vi "SimpleStreamingExample.vi"() -> ()   [LabVIEW 2016]
doc: "This example VI demonstrates the establishment and use of streaming peaks data from Hyperion instruments."
uses:
  h.Library/ACQ/CTL/h.ACQ.PeaksData.ctl
  h.Library/ACQ/CTL/h.ACQ.PeaksWvl.ctl
  h.Library/COMM/CTL/h.COMM.Socket Type.ctl
  h.Library.lvlib
panel:
  out "Peaks Data":T1 {"Peaks Wvls, nm"."Peak Wvls, nm" format="%#_8g"}
  out "Error":errorcluster
  in  "stop":bool
  in  "Data Rate Divider":i32=1 min=1 step=1
  in  "Address":string="10.0.0.55"
  # "Hyperion Simple Streaming Example"
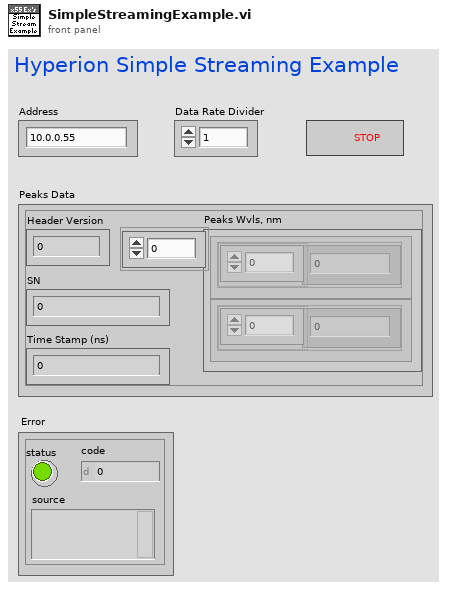
[diagram p1: front panel]
types:
  T1 = typedef "h.Library.lvlib/h.ACQ.PeaksData.ctl" = cluster{"SN":u64, "Time Stamp (ns)":u64, "Header Version":u16, "Peaks Wvls, nm":T2[]}
  T2 = typedef "h.Library.lvlib/h.ACQ.PeaksWvl.ctl" = cluster{"Peak Wvls, nm":dbl[]}
  T3 = typedef "h.Library.lvlib/h.COMM.Socket Type.ctl" = u16
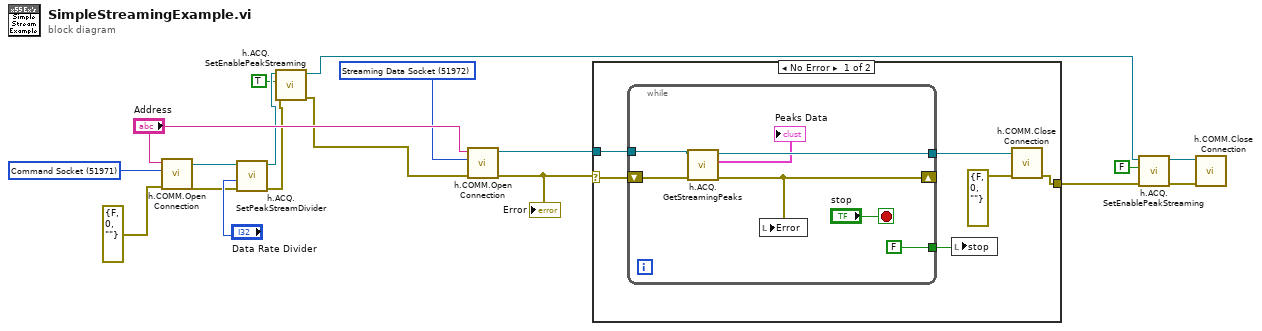
[diagram p0: block diagram]
diagram:
  w10 = T3 51972 items=["Command Socket"=51971, "Streaming Data Socket"=51972] ("Port")
  w11 = T3 51971 items=["Command Socket"=51971, "Streaming Data Socket"=51972] ("Port")
  n1 = call "h.COMM.Open Connection.vi"("error in"=errorcluster {"status"=FALSE, "code"=0, "source"=""}, "Port"=w11, "Address"="Address") -> ("error out"=w15:errorcluster, "Connection ID"=w17:refnum<k5>)  [unwired: 7 in]
  n2 = call "h.ACQ.SetPeakStreamDivider.vi"("error in"=w15, "Data Rate Divider"="Data Rate Divider", "Connection ID In"=w17) -> ("error out"=w7:errorcluster, "Connection ID Out"=w9:refnum<k5>)  [unwired: 7 in]
  n3 = call "h.ACQ.SetEnablePeakStreaming.vi"("error in"=w7, "Enable"=TRUE, "Connection ID in"=w9) -> ("error out"=w6:errorcluster, "Connection ID out"=w3:refnum<k5>)  [unwired: 7 in]
  n4 = call "h.COMM.Open Connection.vi"("error in"=w6, "Port"=w10, "Address"="Address") -> ("error out"=w13:errorcluster, "Connection ID"=w12:refnum<k5>)  [unwired: 7 in]
  "Error" <- w13
  n5 = case shown="No Error" w13 {
    selector: w13 -> [w23 _]
    tunnel: w12 -> [w20 _]
    tunnel: [w19 _] -> w4
    frame No Error {
      n6 = while {
        tunnel: [w30] -> w24
        shift-right: [w28] -> _
        shift-left: w23 -> [w29]
        tunnel: [FALSE ("stop")] -> w21
        tunnel: w20 -> [w25]
        stop <- "stop" stop-if-true
        n7 = call "h.ACQ.GetStreamingPeaks.vi"("error in"=w29, "Connection ID In"=w25) -> ("error out"=w28:errorcluster, "Peaks Data"=→"Peaks Data":T1, "Connection ID Out"=w30:refnum<k5>)  [unwired: 7 in]
        n8 = local write "Error"(w28) -> ()
      }
      n9 = local write "stop"(w21) -> ()
      n10 = call "h.COMM.Close Connection.vi"("error in"=errorcluster {"status"=FALSE, "code"=0, "source"=""}, "Connection ID"=w24) -> ("error out"=w19:errorcluster)  [unwired: 9 in]
    }
    frame Error {
    }
  }
  n11 = call "h.ACQ.SetEnablePeakStreaming.vi"("error in"=w4, "Enable"=FALSE, "Connection ID in"=w3) -> ("error out"=w2:errorcluster, "Connection ID out"=w1:refnum<k5>)  [unwired: 7 in]
  n12 = call "h.COMM.Close Connection.vi"("error in"=w2, "Connection ID"=w1) -> ()  [unwired: 9 in, 1 out]
